vi "Data Source Tree Refresh.vi"(8 "error in (no error)":errorcluster caption="Error In", 9 "GroupInfo In":T3(c390), 10 "Tree In":refnum<vi>, 11 "Data Path":path) -> (0 "error out":errorcluster caption="Error Out", 1 "GroupInfo Out":T3(c390), 3 "Count":string)   [LabVIEW 2020]
uses:
  0007 Controls/005 Data Source Type.ctl
  0007 Controls/002 Group Type.ctl
  <vilib>/Utility/miscctls.llb/LVMapReplaceAction.ctl
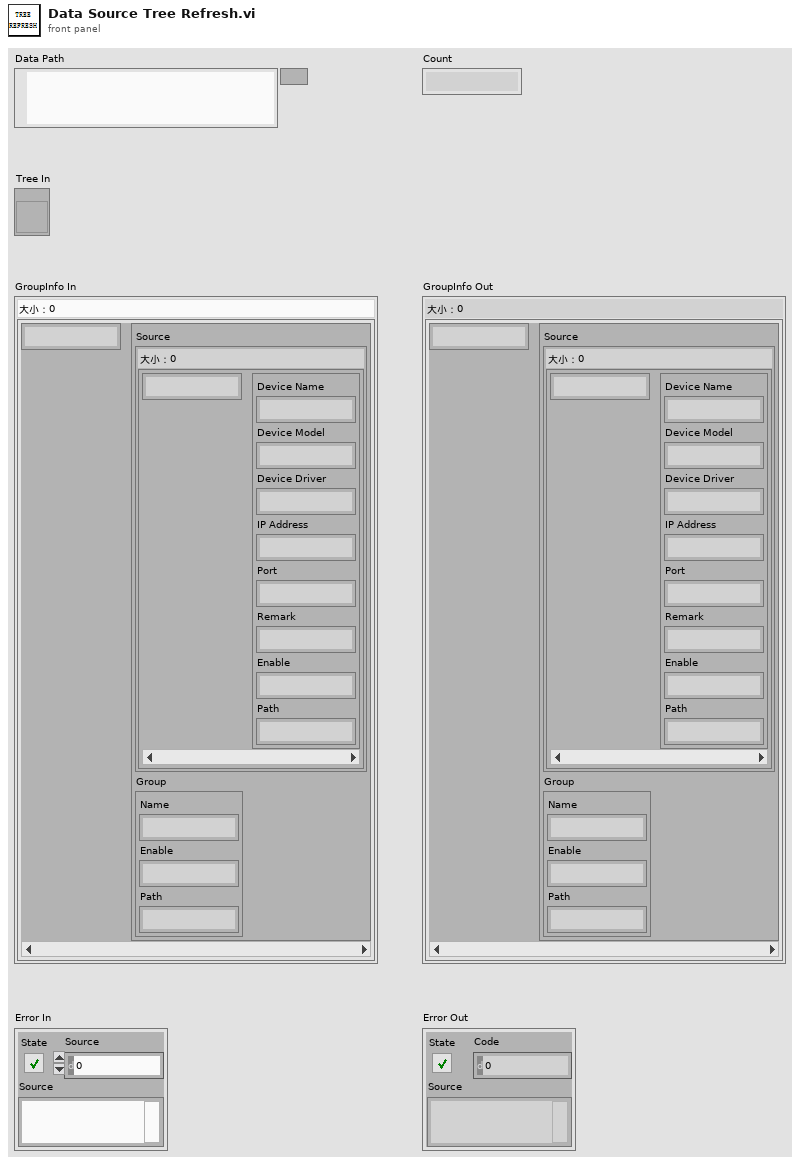
[diagram p1: front panel]
types:
  T1 = typedef "005 Data Source Type.ctl" = cluster{"Device Name":string, "Device Model":string, "Device Driver":string, "IP Address":string, "Port":string, "Remark":string, "Enable":string, "Path":string}
  T2 = typedef "002 Group Type.ctl" = cluster{"Name":string, "Enable":string, "Path":string}
  T3 = map{string, cluster{"Source":map{string, T1}, "Group":T2}}
  T4 = typedef "LVMapReplaceAction.ctl" = enum32{"Modify Entry only if found", "Add or Modify Entry", "Delete Entry"}
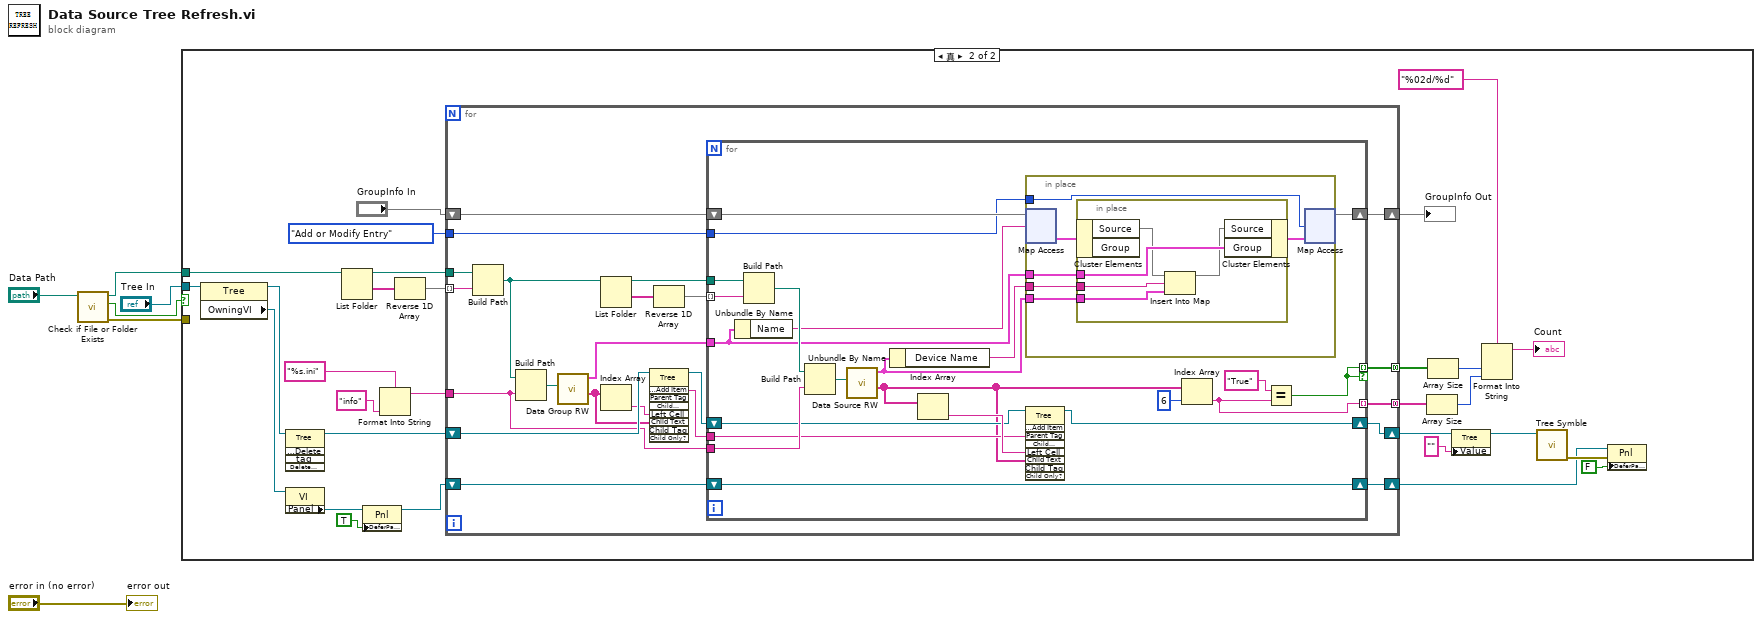
[diagram p0: block diagram]
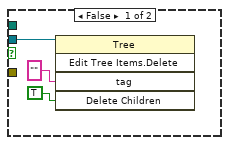
[diagram p2: hidden frame]
diagram:
  n1 = call <vilib>:"Check if File or Folder Exists.vi"("path"="Data Path") -> ("error out"=w2:errorcluster, "file or folder exists?"=w3:bool, "dup path"=w4:path)  [unwired: 8 in]
  n2 = case shown="真" w3 {
    tunnel: w4 -> [_ w11]
    tunnel: w2 -> [_ _]
    tunnel: "Tree In" -> [w9 w10]
    frame False {
      n3 = invoke class="Tree" method="Edit Tree Items.Delete"(reference=w9, "tag"="" ("标识符"), "Delete Children"=TRUE ("删除子项？")) -> ()  [unwired: 2 in, 5 out]
    }
    frame True {
      n4 = property class="Tree"(reference=w10) -> (reference out=w17:refnum<vi>, "OwningVI"=w16:refnum<vi>)  [unwired: 1 in, 1 out]
      n5 = invoke class="Tree" method="Edit Tree Items.Delete"(reference=w17) -> (reference out=w35:refnum<vi>)  [unwired: 4 in, 4 out]
      n6 = property class="VI"(reference=w16) -> ("Panel"=w29:refnum<vi>)  [unwired: 1 in, 2 out]
      n7 = List Folder(path=w11) -> (path out=w38:path, folder names=w37:string[])  [unwired: 3 in, 2 out]
      n8 = property class="Pnl"(reference=w29, "DeferPanUpdts"=TRUE ("延迟前面板更新")) -> (reference out=w27:refnum<vi>)  [unwired: 1 in, 1 out]
      n9 = Format Into String(format string="%s.ini" ("格式字符串"), "info" ("输入 1")) -> (resulting string=w33:string)  [unwired: 2 in, 1 out]
      n10 = Reverse 1D Array(array=w37) -> (reversed array=w36:string[])
      n11 = for {
        tunnel: w38 -> [w60]
        tunnel: w36 -> [w58] mode=indexing
        shift-right: [w52] -> w30
        shift-left: w35 -> [w59]
        shift-right: [w47] -> w18
        shift-left: w27 -> [w48]
        tunnel: [w46] -> w24 mode=concatenating
        tunnel: [w45] -> w23 mode=concatenating
        tunnel: w33 -> [w51]
        shift-right: [w41] -> w13
        shift-left: "GroupInfo In" -> [w42]
        tunnel: LVMapReplaceAction."Add or Modify Entry" ("操作") -> [w40]
        n12 = Build Path(base path=w60, name or relative path=w58) -> (appended path=w56:path)
        n13 = Build Path(base path=w56, name or relative path=w51) -> (appended path=w44:path)
        n14 = call "Data Group RW.vi"("Source Path"=w44) -> ("Data"=w43:string[], "Group Type Out"=w39:T2)  [unwired: 7 in, 2 out]
        n15 = List Folder(path=w56) -> (path out=w54:path, folder names=w57:string[])  [unwired: 3 in, 2 out]
        n16 = Index Array(array=w43) -> (element=w49:string)  [unwired: 1 in]
        n17 = invoke class="Tree" method="Edit Tree Items.Add Item"(reference=w59, "Left Cell"=w49, "Child Text"=w43) -> (reference out=w53:refnum<vi>, "Edit Tree Items:Add Item"=w50:string)  [unwired: 6 in, 7 out]
        n18 = Reverse 1D Array(array=w57) -> (reversed array=w55:string[])
        n19 = for {
          tunnel: w55 -> [w81] mode=indexing
          tunnel: w54 -> [w82]
          shift-right: [w78] -> w52
          shift-left: w53 -> [w75]
          tunnel: w50 -> [w76]
          shift-right: [w74] -> w47
          shift-left: w48 -> [w74]
          tunnel: [w72] -> w46 mode=indexing
          tunnel: [w70] -> w45 mode=indexing if=w70
          tunnel: w51 -> [w79]
          shift-right: [w66] -> w41
          shift-left: w42 -> [w67]
          tunnel: w40 -> [w65]
          tunnel: w39 -> [w61]
          n20 = Unbundle By Name(w61) -> ("Name"=w62:string)
          n21 = Build Path(base path=w82, name or relative path=w81) -> (appended path=w80:path)
          n22 = Build Path(base path=w80, name or relative path=w79) -> (appended path=w68:path)
          n23 = call "Data Source RW.vi"("Source Path"=w68) -> ("Data"=w69:string[], "Data Type Out"=w63:T1)  [unwired: 7 in, 2 out]
          n24 = Unbundle By Name(w63) -> ("Device Name"=w64:string)
          n25 = Index Array(array=w69) -> (element=w77:string)  [unwired: 1 in]
          n26 = in-place {
            in-place-border: w61 -> [w87]
            in-place-border: w64 -> [w85]
            in-place-border: w65 -> [w84]
            in-place-border: w63 -> [w83]
            n27 = in-place-map #1(w67, w62) -> (w88:cluster{"Source":map{string, T1}, "Group":T2})  [unwired: 1 in, 1 out]
            n28 = in-place {
              in-place-border: w87 -> [w93]
              in-place-border: w85 -> [w89]
              in-place-border: w83 -> [w90]
              n29 = in-place-cluster #2(w88) -> ("Source"=w92:map{string, T1})  [unwired: 1 out]
              n30 = Insert Into Map(map in=w92, key=w89, value=w90) -> (map out=w91:map{string, T1})  [unwired: 2 out]
              n31 = in-place-cluster #2("Source"=w91, "Group"=w93) -> (w86:cluster{"Source":map{string, T1}, "Group":T2})
            }
            n32 = in-place-map #1(w86, w84) -> (w66:T3)  [unwired: 2 out]
          }
          n33 = invoke class="Tree" method="Edit Tree Items.Add Item"(reference=w75, "Parent Tag"=w76, "Left Cell"=w77, "Child Text"=w69) -> (reference out=w78:refnum<vi>)  [unwired: 5 in, 8 out]
          n34 = Index Array(array=w69, index=6 ("索引")) -> (element=w72:string)
          n35 = Equal?(x="True", y=w72) -> (x = y?=w70:bool)
        }
      }
      "GroupInfo Out" <- w13
      n36 = Array Size(array=w24) -> (size(s)=w20:i32)
      n37 = Array Size(array=w23) -> (size(s)=w21:i32)
      n38 = property class="Tree"(reference=w30, "Value"="") -> (reference out=w25:refnum<vi>)  [unwired: 1 in, 1 out]
      n39 = Format Into String(format string="%02d/%d", w21, w20) -> (resulting string=→"Count":string)  [unwired: 2 in, 1 out]
      n40 = call "Tree Symble.vi"("Tree In"=w25) -> ("error out"=w19:errorcluster)  [unwired: 9 in, 1 out]
      n41 = property class="Pnl"(reference=w18, error in=w19, "DeferPanUpdts"=FALSE ("延迟前面板更新")) -> ()  [unwired: 2 out]
    }
  }
  "error out" <- "error in (no error)"
